vi "Write Topologies.vi"(10 "Topologies":T1[](array[typedef]), 11 "SLSC Switch in":refnum<class "SLSC Switch.lvclass">) -> (3 "SLSC Switch out":refnum<class "SLSC Switch.lvclass">)   [LabVIEW 2015, in "SLSC Switch.lvclass"]
uses:
  SLSC Switch.lvclass
  Controls/Topology.ctl
  SLSC Switch.lvclass/SLSC Switch.ctl
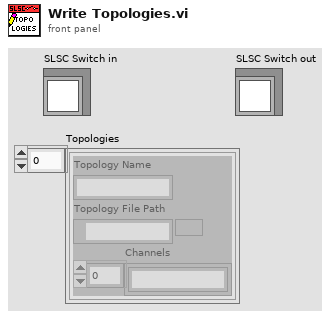
[diagram p1: front panel]
types:
  T1 = typedef "SLSC Switch.lvclass/Topology.ctl" = cluster{"Topology Name":string, "Topology File Path":path, "Channels":string[]}
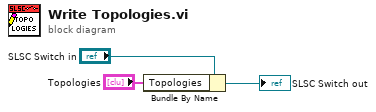
[diagram p0: block diagram]
diagram:
  n1 = Bundle By Name(cluster="SLSC Switch in", "Topologies"="Topologies") -> (→"SLSC Switch out":refnum<class "SLSC Switch.lvclass">)
